vi "Air Puff.vi"() -> ()   [LabVIEW 2012]
panel:
  in  "#Cycle":i32=2
  out "Cycle#":i32=2
  in  "Post-Stim Time (s)":dbl=5.0
  in  "Stim Time (s)":dbl=2.0
  out "air puff":bool[](array[boolean])
  in  "Pre-Stim Time (s)":dbl=5.0
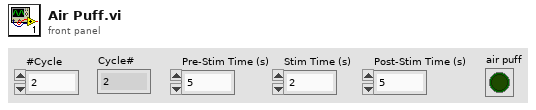
[diagram p1: front panel]
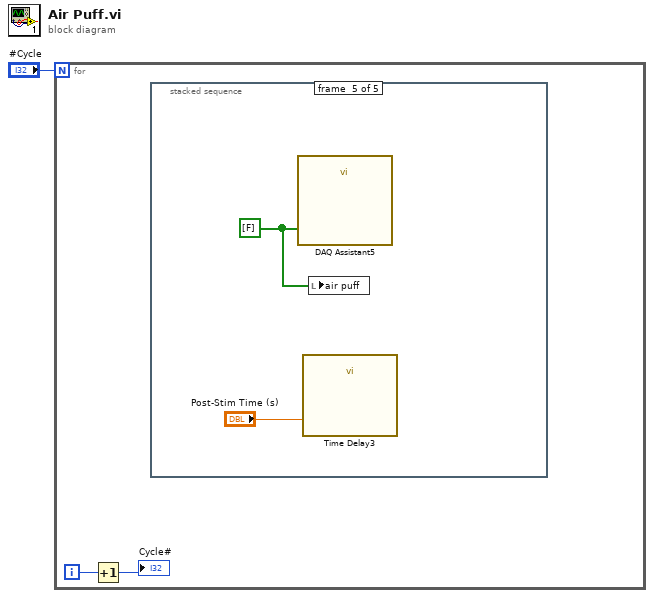
[diagram p0: block diagram]
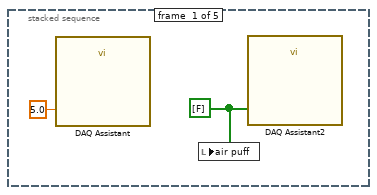
[diagram p2: hidden frame]
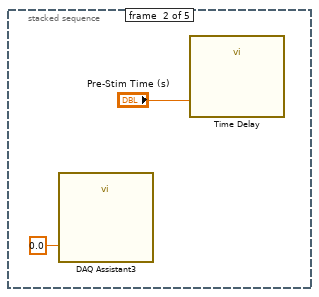
[diagram p3: hidden frame]
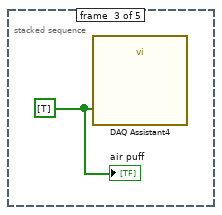
[diagram p4: hidden frame]
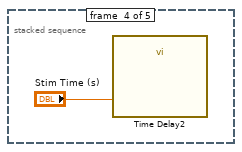
[diagram p5: hidden frame]
diagram:
  n1 = for {
    N: "#Cycle" -> [_]
    i -> [w3]
    n2 = Increment(x=w3) -> (x+1=→"Cycle#":i32)
    n3 = stacked-sequence {
      frame #0 {
        w4 = bool[] [FALSE] ("data")
        n4 = call "DAQ Assistant"("data"=5.0) -> ()  [unwired: 17 in, 2 out]
        n5 = local write "air puff"(w4) -> ()
        n6 = call "DAQ Assistant2"("data"=w4) -> ()  [unwired: 17 in, 2 out]
      }
      frame #1 {
        n7 = call "DAQ Assistant3"("data"=0.0) -> ()  [unwired: 17 in, 2 out]
        n8 = call "Time Delay"("Delay Time (s)"="Pre-Stim Time (s)") -> ()  [unwired: 10 in, 1 out]
      }
      frame #2 {
        w8 = bool[] [TRUE] ("data")
        n9 = call "DAQ Assistant4"("data"=w8) -> ()  [unwired: 17 in, 2 out]
        "air puff" <- w8
      }
      frame #3 {
        n10 = call "Time Delay2"("Delay Time (s)"="Stim Time (s)") -> ()  [unwired: 10 in, 1 out]
      }
      frame #4 {
        w10 = bool[] [FALSE] ("data")
        n11 = call "DAQ Assistant5"("data"=w10) -> ()  [unwired: 17 in, 2 out]
        n12 = call "Time Delay3"("Delay Time (s)"="Post-Stim Time (s)") -> ()  [unwired: 10 in, 1 out]
        n13 = local write "air puff"(w10) -> ()
      }
    }
  }
